vi "Nikhil 3rd year usb new.vi"() -> ()   [LabVIEW 2014]
panel:
  out "Amplitude 2":dbl
  out "Boolean 2":bool
  out "Filtered Signal 4":dynamicdata(graph) caption="Filtered Signal"
  out "Amplitude":dbl
  out "Result 3":dbl
  out "Result 2":dbl
  out "Result":dynamicdata(graph)
  out "Filtered Signal 3":dynamicdata(graph) caption="Filtered Signal"
  out "Filtered Signal 2":dynamicdata(graph) caption="Filtered Signal"
  out "Filtered Signal":dynamicdata(graph)
  in  "stop (F)":bool
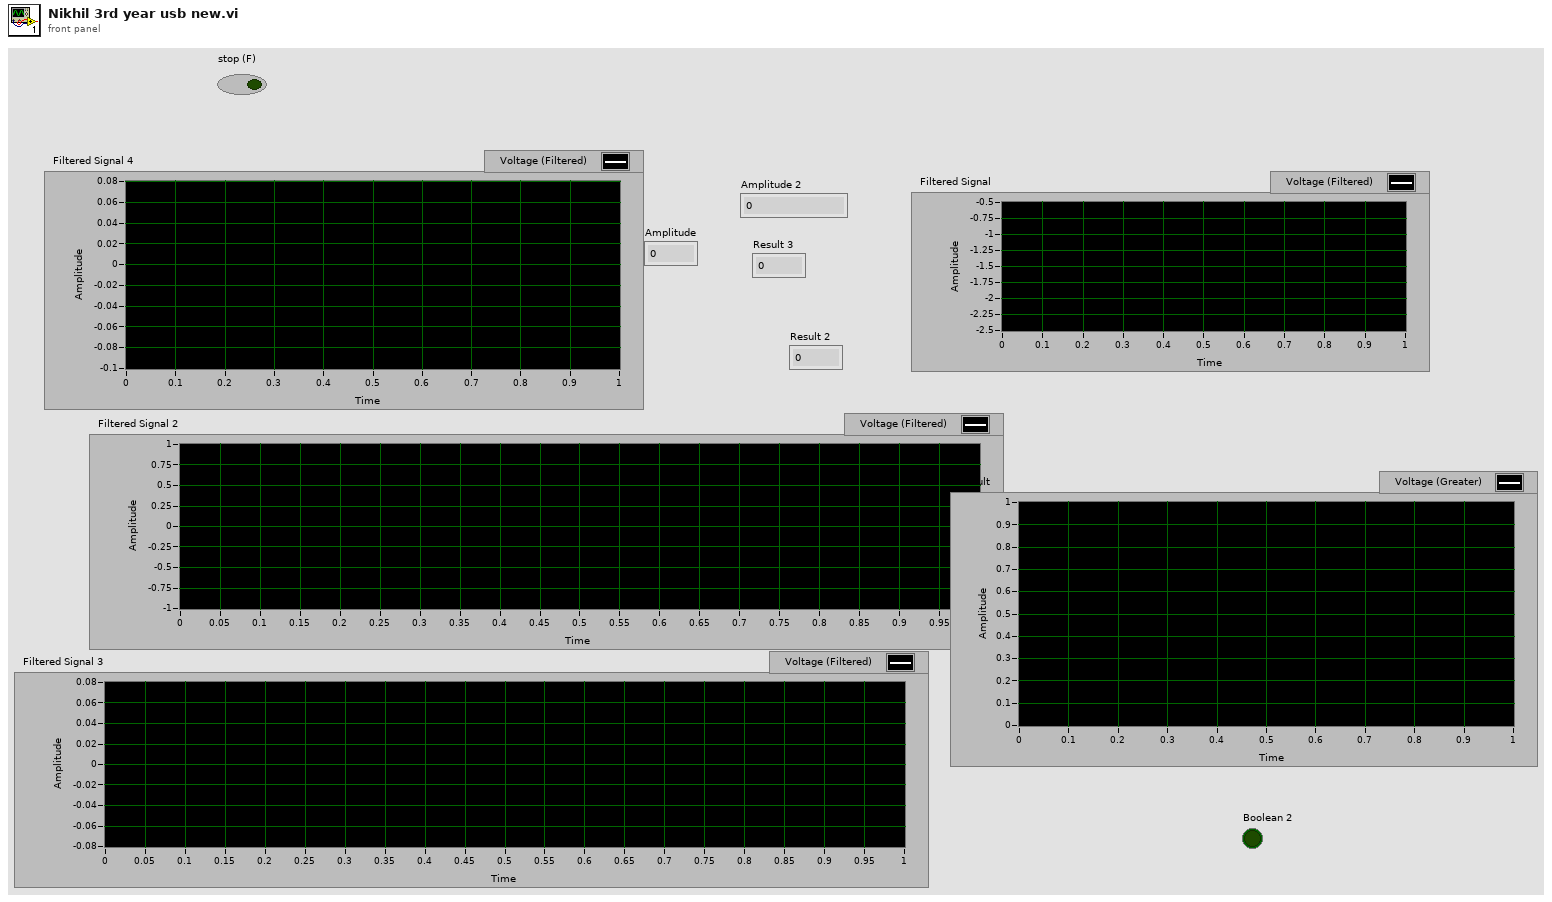
[diagram p1: front panel]
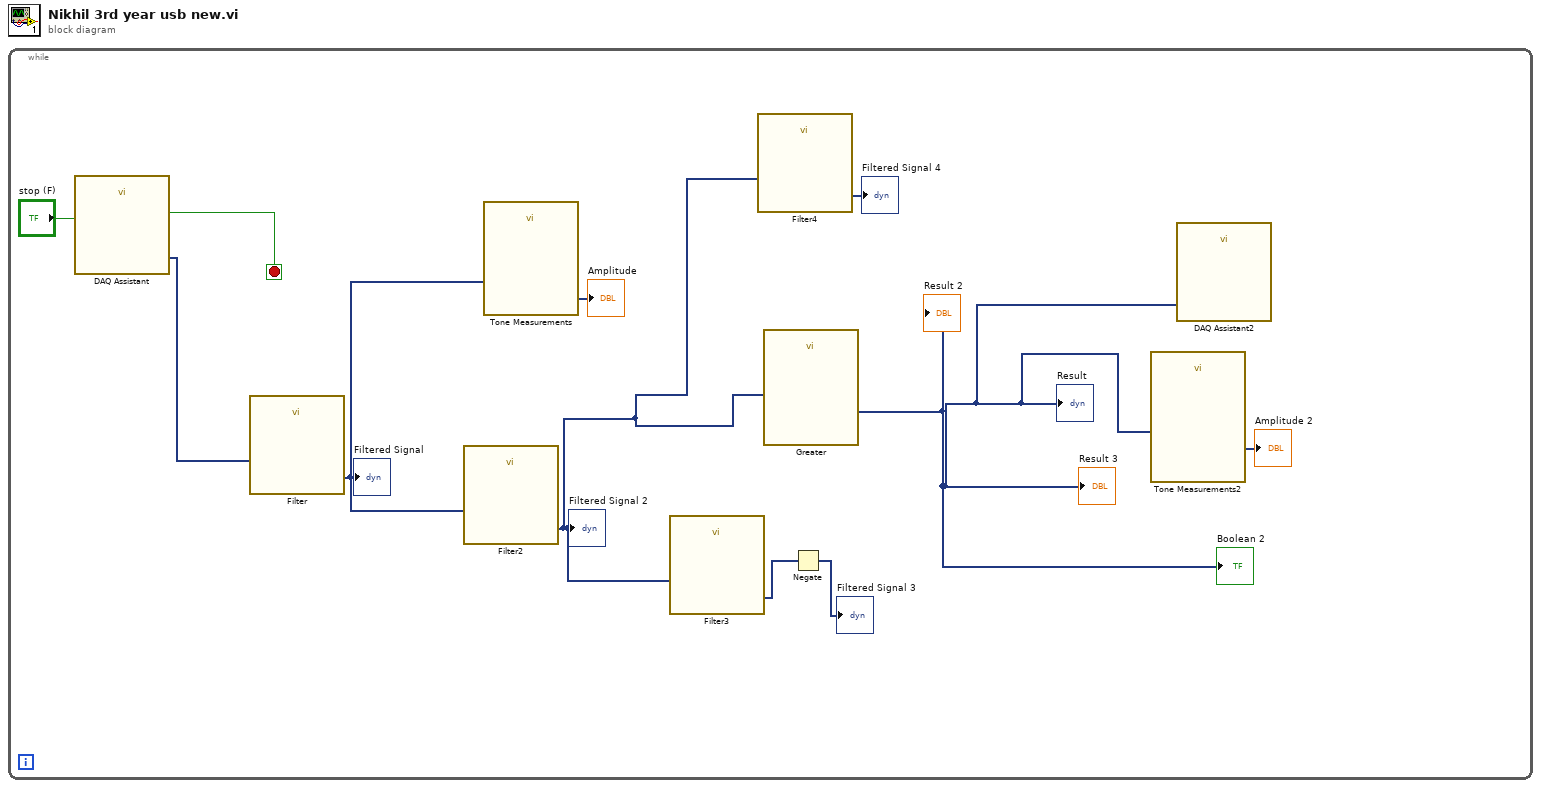
[diagram p0: block diagram]
diagram:
  n1 = while {
    stop <- w10 stop-if-true
    n2 = call "DAQ Assistant"("stop (F)"="stop (F)") -> ("data"=w8:dynamicdata, "stopped"=w10:bool)  [unwired: 15 in, 2 out]
    n3 = call "Filter"("Signal"=w8) -> ("Filtered Signal"=w3:dynamicdata)  [unwired: 9 in, 1 out]
    "Filtered Signal" <- w3
    n4 = call "Filter2"("Signal"=w3) -> ("Filtered Signal"=w1:dynamicdata)  [unwired: 9 in, 1 out]
    "Filtered Signal 2" <- w1
    n5 = call "Tone Measurements"("Signals"=w3) -> ("Amplitude"=→"Amplitude":dynamicdata)  [unwired: 9 in, 1 out]
    n6 = call "Filter3"("Signal"=w1) -> ("Filtered Signal"=w9:dynamicdata)  [unwired: 9 in, 1 out]
    n7 = call "Filter4"("Signal"=w1) -> ("Filtered Signal"=→"Filtered Signal 4":dynamicdata)  [unwired: 9 in, 1 out]
    n8 = call "Greater"("Operand 1"=w1) -> ("Result"=w2:dynamicdata)  [unwired: 9 in, 1 out]
    "Result" <- w2
    "Result 2" <- w2
    "Result 3" <- w2
    "Boolean 2" <- w2
    n9 = Negate(x=w9) -> (-x=→"Filtered Signal 3":dynamicdata)
    n10 = call "Tone Measurements2"("Signals"=w2) -> ("Amplitude"=→"Amplitude 2":dynamicdata)  [unwired: 8 in, 2 out]
    n11 = call "DAQ Assistant2"("data"=w2) -> ()  [unwired: 16 in, 3 out]
  }
